vi "Looped_Grid_V1.vi"() -> ()   [LabVIEW 2014]
uses:
  <userlib>/Nanonis Prog Interface V5/Nanonis Prog Interface.lvlib
panel:
  in  "String":string
  in  "Numeric":i32
  out "set value":dbl format="%#_6p"
  out "next value":dbl=2e-10 format="%#_6p"
  out "waited:":i32=20000 format="%.0p"
  out "Grid Running?":bool=TRUE
  in  "External VI path":path=path "D:/Scripts/VIs/Topo & GridSpectr_DriftCorrection_zSpec_v19.vi"
  in  "engage":bool=TRUE
  in  "Control Name":string="STS z offset"
  # "Zero is \"0\""
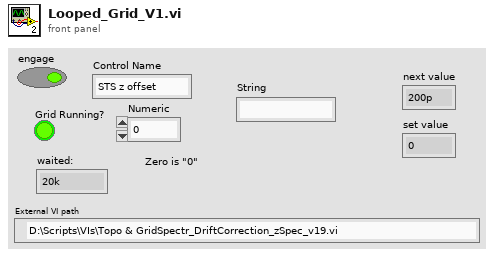
[diagram p1: front panel]
types:
  T1 = enum16{"Header", "TOPO", "STS", "GRID", "GRIDCloud"}
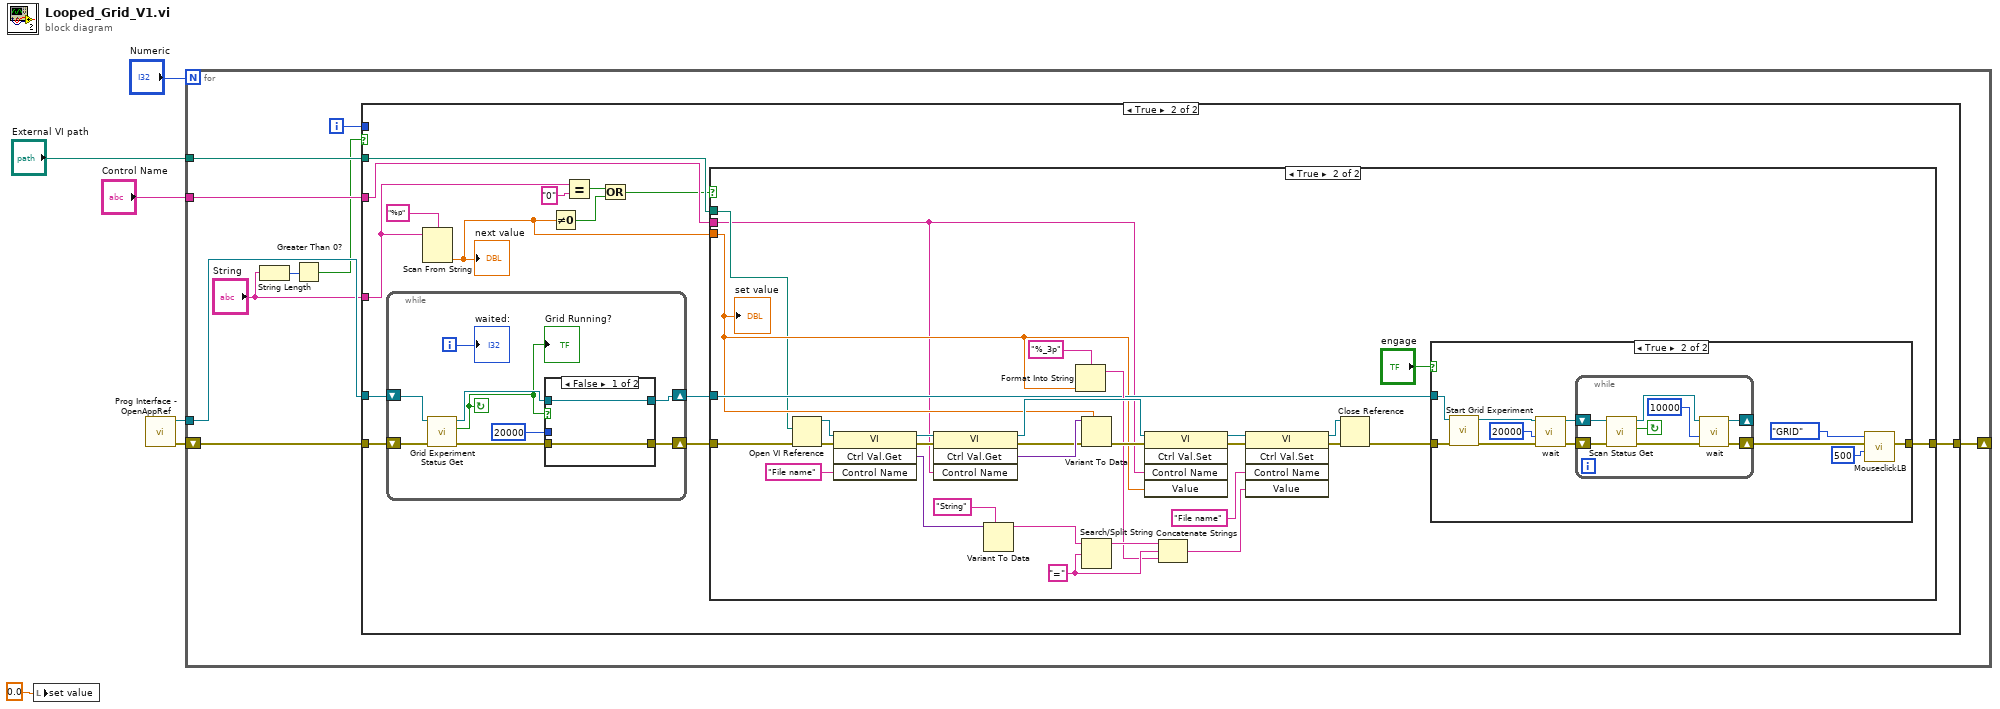
[diagram p0: block diagram]
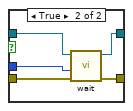
[diagram p5: hidden frame]
diagram:
  n1 = local write "set value"(0.0 ("set value")) -> ()
  n2 = call <userlib>:"Prog Interface - OpenAppRef.vi"() -> ("Error out"=w6:errorcluster, "Application reference"=w5:refnum<vi>)  [unwired: 6 in]
  n3 = for {
    N: "Numeric" -> [_]
    tunnel: w5 -> [w14]
    tunnel: "External VI path" -> [w12]
    tunnel: "Control Name" -> [w11]
    shift-right: [w10] -> _
    shift-left: w6 -> [w15]
    i -> [w13]
    n4 = String Length(string="String") -> (length=w9:i32)
    n5 = Greater Than 0?(x=w9) -> (x > 0?=w8:bool)
    n6 = case shown="True" w8 {
      tunnel: w15 -> [w16 w30]
      tunnel: w14 -> [_ w29]
      tunnel: w13 -> [_ _]
      tunnel: "String" -> [_ w23]
      tunnel: w12 -> [_ w20]
      tunnel: w11 -> [_ w19]
      tunnel: [w16 w18] -> w10
      frame False {
      }
      frame True {
        n7 = while {
          shift-right: [w87] -> w28
          shift-left: w29 -> [w89]
          shift-right: [w86] -> w27
          shift-left: w30 -> [w90]
          i -> [w83]
          stop <- w82 continue-if-true
          n8 = call <userlib>:"Grid Experiment Status Get.vi"("error in (no error)"=w90, "Application ref in"=w89) -> ("error out"=w85:errorcluster, "Running?"=w82:bool, "Application ref out"=w88:refnum<vi>)  [unwired: 7 in]
          "Grid Running?" <- w82
          n9 = case shown="False" w82 {
            tunnel: w88 -> [w92 w97]
            tunnel: [w92 w96] -> w87
            tunnel: [w91 w95] -> w86
            tunnel: w85 -> [w91 w94]
            tunnel: u32 20000 ("milliseconds to wait") -> [_ w93]
            frame False {
            }
            frame True {
              n10 = call "wait.vi"("error in"=w94, "milliseconds to wait"=w93, "application reference in"=w97) -> ("error out"=w95:errorcluster, "application reference out"=w96:refnum<vi>)  [unwired: 7 in]
            }
          }
          "waited:" <- w83
        }
        n11 = Scan From String(format string="%p", input string=w23) -> (output 1=w21:dbl)  [unwired: 3 in, 3 out]
        "next value" <- w21
        n12 = Not Equal To 0?(x=w21) -> (x != 0?=w22:bool)
        n13 = Equal?(x=w23, y="0") -> (x = y?=w24:bool)
        n14 = Or(x=w24, y=w22) -> (x .or. y?=w17:bool)
        n15 = case shown="True" w17 {
          tunnel: w28 -> [_ w37]
          tunnel: w27 -> [w31 w36]
          tunnel: w21 -> [_ w35]
          tunnel: w20 -> [_ w34]
          tunnel: w19 -> [_ w33]
          tunnel: [w31 w32] -> w18
          frame False {
          }
          frame True {
            w42 = "=" ("search string")
            n16 = Open VI Reference(vi path=w34, error in (no error)=w36) -> (vi reference=w56:refnum<vi>, error out=w55:errorcluster)  [unwired: 4 in]
            n17 = invoke class="VI" method="Ctrl Val.Get"(reference=w56, error in=w55, "Control Name"="File name") -> (reference out=w54:refnum<vi>, error out=w53:errorcluster, "Get Control Value Variant"=w46:variant)  [unwired: 1 in, 1 out]
            n18 = invoke class="VI" method="Ctrl Val.Get"(reference=w54, error in=w53, "Control Name"=w33) -> (reference out=w61:refnum<vi>, error out=w59:errorcluster, "Get Control Value Variant"=w60:variant)  [unwired: 1 in, 1 out]
            n19 = Variant To Data(type="String" ("Control Name"), Variant=w46) -> (data=w44:string)  [unwired: 1 in, 1 out]
            n20 = Format Into String(format string="%_3p", w35) -> (resulting string=w40:string)  [unwired: 2 in, 1 out]
            n21 = Variant To Data(error in=w59, type=w35, Variant=w60) -> (error out=w58:errorcluster)  [unwired: 1 out]
            n22 = Search/Split String(string=w44, search string/char (-)=w42) -> (substring before match=w41:string)  [unwired: 1 in, 2 out]
            n23 = invoke class="VI" method="Ctrl Val.Set"(reference=w61, error in=w58, "Control Name"=w33, "Value"=w35) -> (reference out=w52:refnum<vi>, error out=w51:errorcluster)  [unwired: 1 in, 3 out]
            n24 = Concatenate Strings(w41, w42, w40) -> (w39:string)
            n25 = invoke class="VI" method="Ctrl Val.Set"(reference=w52, error in=w51, "Control Name"="File name", "Value"=w39) -> (reference out=w50:refnum<vi>, error out=w49:errorcluster)  [unwired: 1 in, 3 out]
            n26 = Close Reference(reference=w50, error in (no error)=w49) -> (error out=w57:errorcluster)
            n27 = case shown="True" "engage" {
              tunnel: w57 -> [w62 w73]
              tunnel: w37 -> [_ w72]
              tunnel: [w62 w65] -> w32
              frame False {
              }
              frame True {
                n28 = call <userlib>:"Start Grid Experiment.vi"("Application ref in"=w72, "error in (no error)"=w73) -> ("Application ref out"=w71:refnum<vi>, "error out"=w70:errorcluster)  [unwired: 16 in]
                n29 = call "wait.vi"("error in"=w70, "milliseconds to wait"=u32 20000, "application reference in"=w71) -> ("error out"=w69:errorcluster, "application reference out"=w68:refnum<vi>)  [unwired: 7 in]
                n30 = while {
                  shift-right: [w74] -> w66
                  shift-left: w69 -> [w80]
                  shift-right: [w75] -> _
                  shift-left: w68 -> [w81]
                  stop <- w79 continue-if-true
                  n31 = call <userlib>:"Scan Status Get.vi"("error in (no error)"=w80, "Application ref in"=w81) -> ("error out"=w78:errorcluster, "Scanning?"=w79:bool, "Application ref out"=w77:refnum<vi>)  [unwired: 6 in]
                  n32 = call "wait.vi"("error in"=w78, "milliseconds to wait"=u32 10000, "application reference in"=w77) -> ("error out"=w74:errorcluster, "application reference out"=w75:refnum<vi>)  [unwired: 7 in]
                }
                n33 = call "MouseclickLB.vi"("nMilliseconds"=500, "error in (no error)"=w66, "Click"=T1."GRID") -> ("error out"=w65:errorcluster)  [unwired: 8 in]
              }
            }
            "set value" <- w35
          }
        }
      }
    }
  }
